vi "Phaeron App Template.vi"() -> ()   [LabVIEW 2013]
uses:
  <vilib>/Utility/miscctls.llb/LVPointTypeDef.ctl
  <vilib>/NI/AMC/Read Next Message.vi
  <vilib>/NI/AMC/Create Single Message.vi
  <vilib>/NI/AMC/Update Message Routing Info.vi
  <vilib>/NI/AMC/Read Termination Message.vi
  <vilib>/NI/AMC/Send Message.vi
  <vilib>/NI/AMC/Globals.vi
  <vilib>/NI/AMC/AMC.lvlib
  <vilib>/Phaeron, Inc/JSON/LV JSON.lvlib
panel:
  in  "Stop Loops":bool
  in  "Exit":bool
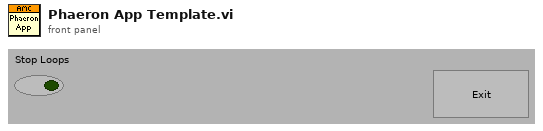
[diagram p1: front panel]
types:
  T1 = typedef "AMC.lvlib/Message Queue.ctl" = refnum<queue>
  T2 = typedef "LVPointTypeDef.ctl" = cluster{"Horizontal":i16, "Vertical":i16}
  T3 = typedef "LVRectTypeDef.ctl" = cluster{"Left":i16, "Top":i16, "Right":i16, "Bottom":i16}
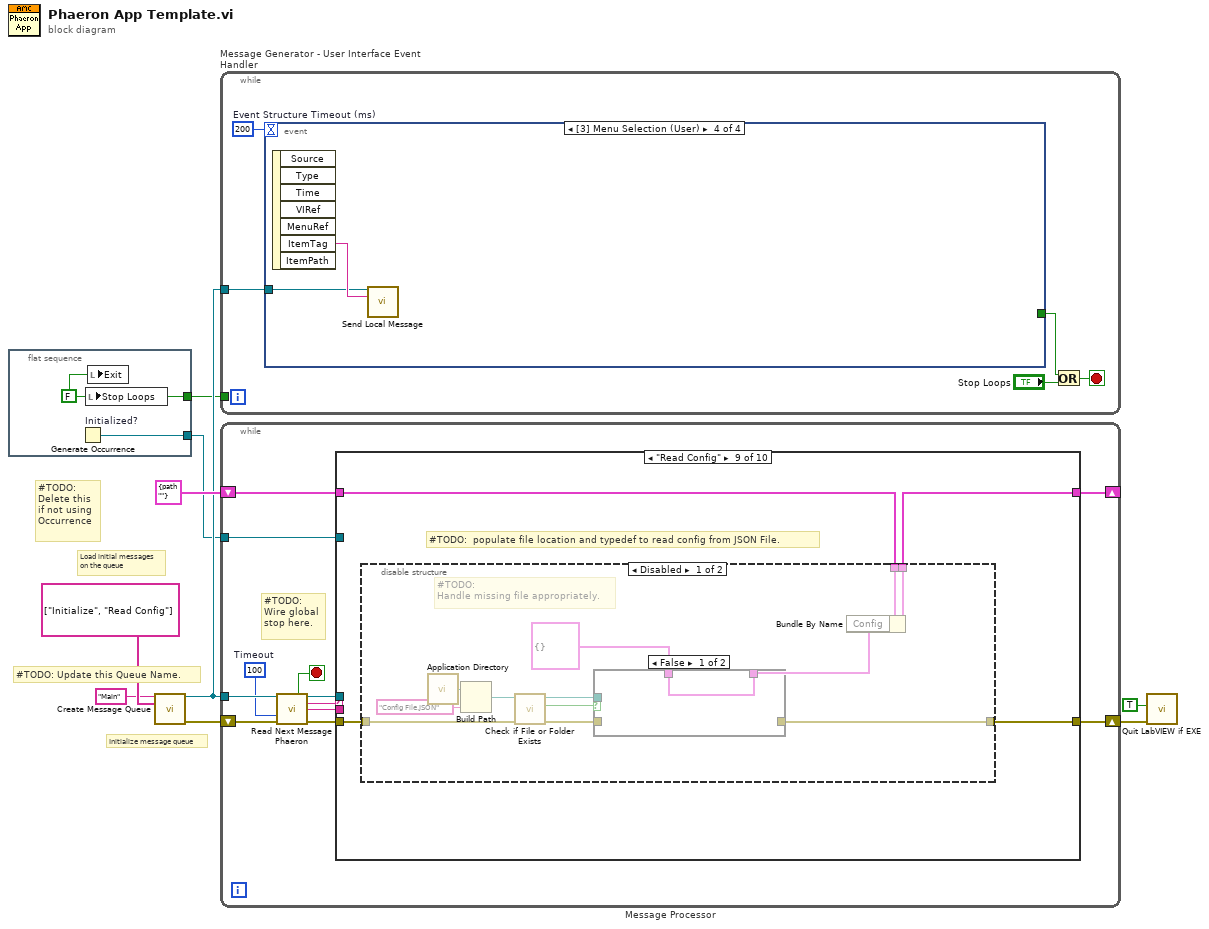
[diagram p0: block diagram]
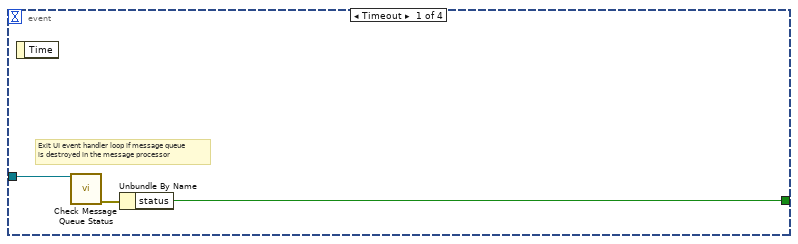
[diagram p2: hidden frame]
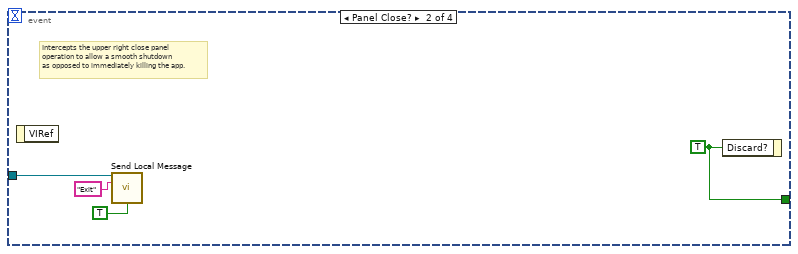
[diagram p3: hidden frame]
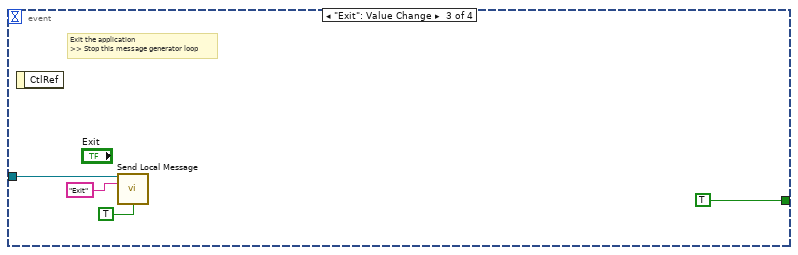
[diagram p4: hidden frame]
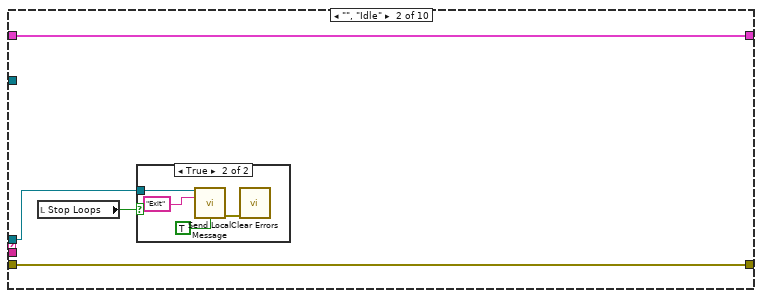
[diagram p6: hidden frame]
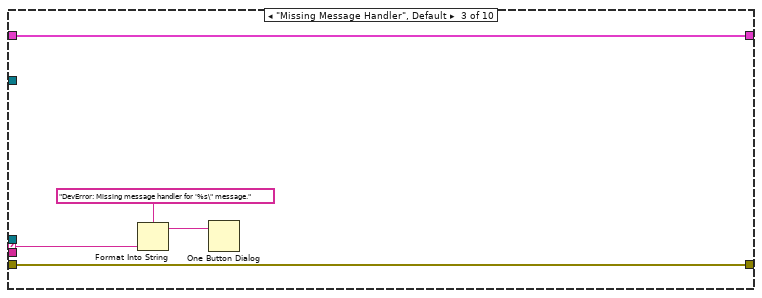
[diagram p8: hidden frame]
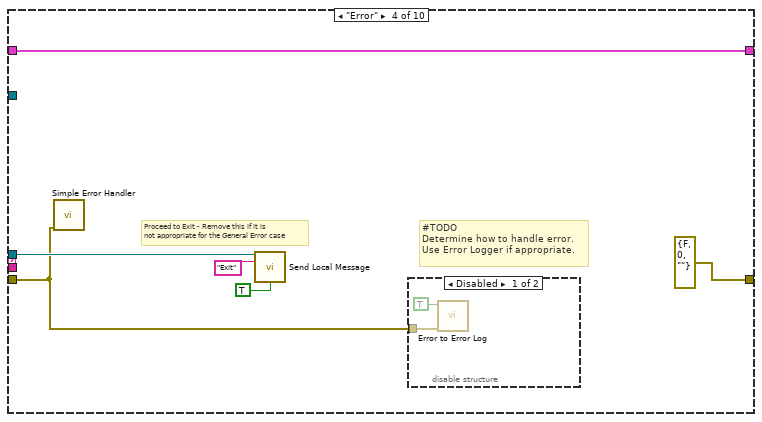
[diagram p9: hidden frame]
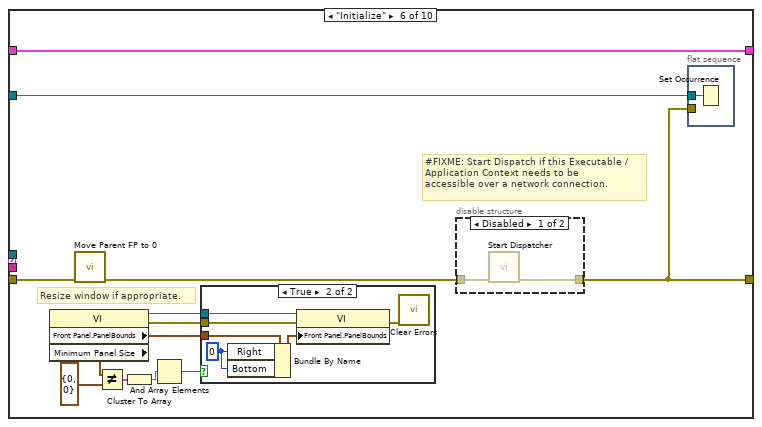
[diagram p12: hidden frame]
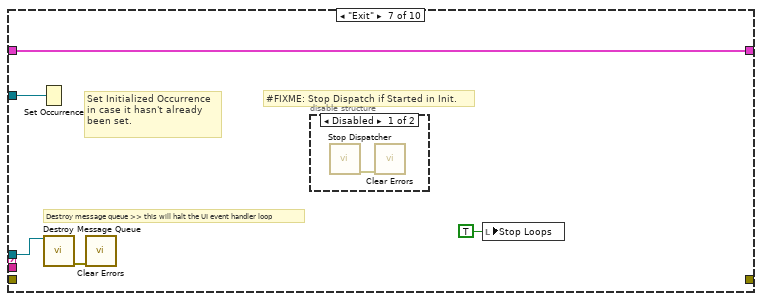
[diagram p15: hidden frame]
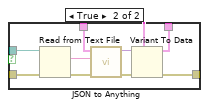
[diagram p18: hidden frame]
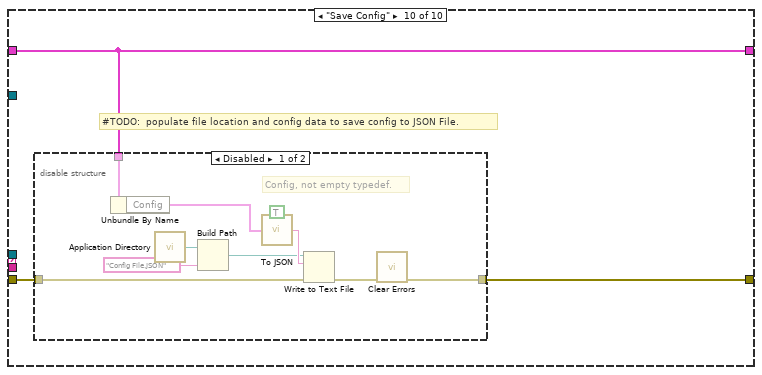
[diagram p20: hidden frame]
diagram:
  # "#TODO:\nDelete this\nif not using\nOccurrence"
  # "#TODO: Update this Queue Name."
  # "Initialize message queue"
  # "Load initial messages\non the queue"
  n1 = flat-sequence {
    tunnel: [w10] -> w4
    tunnel: [w11] -> w1
    frame #0 {
      w10 = FALSE ("Stop Loops")
      n2 = Generate Occurrence "Initialized?"() -> (w11:refnum<k4>)
      n3 = local write "Stop Loops"(w10) -> ()
      n4 = local write "Exit"(w10) -> ()
    }
  }
  n5 = call <vilib>:"Create Message Queue.vi"("message queue name"="Main", "initial message names"=string[] ["Initialize", "Read Config"]) -> ("message queue out"=w7:T1, "error out"=w8:errorcluster)  [unwired: 12 in]
  n6 = while "Message Generator - User Interface Event Handler" {
    tunnel: w7 -> [w14]
    tunnel: w4 -> [_]
    stop <- w13 stop-if-true
    w16 = 200  # Event Structure Timeout (ms)
    n7 = event shown="[3] Menu Selection (User)" {
      selector: _ -> [_ _ _ _]
      dyn-events: _ -> [_ _ _ _]
      timeout: w16 -> [_ _ _ _]
      tunnel: [w17 w20 TRUE ("Discard?") _] -> w15
      tunnel: w14 -> [w18 w22 w25 w28]
      event Timeout {
        # "Exit UI event handler loop if message queue\nis destroyed in the message processor"
        n8 = event-data() -> ()  [unwired: 2 out]
        n9 = call <vilib>:"Check Message Queue Status.vi"("message queue in"=w18) -> ("error out"=w19:errorcluster)  [unwired: 10 in, 4 out]
        n10 = Unbundle By Name(w19) -> ("status"=w17:bool)
      }
      event Panel Close? {
        w20 = TRUE ("Discard?")
        # "Intercepts the upper right close panel\noperation to allow a smooth shutdown\nas opposed to immediately killing the app."
        n11 = event-data() -> ()  [unwired: 2 out]
        n12 = call <vilib>:"Send Local Message.vi"("message queue in"=w22, "message name"="Exit", "priority message (F)"=TRUE) -> ()  [unwired: 10 in, 3 out]
        n13 = event-data("Discard?"=w20) -> ()  [unwired: 1 in, 1 out]
      }
      event "Exit": Value Change {
        # "Exit the application\n>> Stop this message generator loop"
        n14 = event-data() -> ()  [unwired: 2 out]
        n15 = call <vilib>:"Send Local Message.vi"("message queue in"=w25, "message name"="Exit", "priority message (F)"=TRUE) -> ()  [unwired: 10 in, 3 out]
      }
      event Menu Selection (User) {
        n16 = event-data() -> ("ItemTag"=w29:string)  [unwired: 7 out]
        n17 = call <vilib>:"Send Local Message.vi"("message queue in"=w28, "message name"=w29) -> ()  [unwired: 11 in, 3 out]
      }
    }
    n18 = Or(x=w15, y="Stop Loops") -> (x .or. y?=w13:bool)
  }
  n19 = while "Message Processor" {
    shift-left: w8 -> [w35]
    shift-right: [w39] -> w3
    tunnel: w7 -> [w36]
    shift-left: cluster{"CurrentFile":path} {"CurrentFile"=path ""} ("State Variables") -> [w41]
    shift-right: [w40] -> _
    tunnel: w1 -> [w30]
    stop <- w38 stop-if-true
    w31 = 100  # Timeout
    # "#TODO:\nWire global\nstop here."
    n20 = call "Read Next Message Phaeron.vi"("message queue in"=w36, "timeout (1 ms)"=w31, "error in"=w35) -> ("exit process?"=w38:bool, "message queue out"=w37:T1, "message name"=w33:string, "message value"=w32:string, "error out"=w34:errorcluster)  [unwired: 5 in, 3 out]
    n21 = case shown="\"Read Config\"" w33 {
      selector: w33 -> [_ _ w54 _ _ _ _ _ _ _]
      tunnel: [w43 w47 w56 w62 w66 w79 w94 w97 w98 w126] -> w40
      tunnel: w41 -> [w43 w47 w56 w62 w66 w79 w94 w97 w99 w126]
      tunnel: w37 -> [_ w45 _ w60 _ _ w93 _ _ _]
      tunnel: w34 -> [w42 w46 w55 w57 w65 w78 _ w96 w101 w128]
      tunnel: [w42 w46 w55 errorcluster {"status"=FALSE, "code"=0, "source"=""} ("error out") w65 w75 _ w96 w100 w127] -> w39
      tunnel: w32 -> [_ _ _ _ _ _ _ _ _ _]
      tunnel: w30 -> [_ _ _ _ _ w76 w90 _ _ _]
      frame "---------- Framework Operations ----------" {
      }
      frame "", "Idle" {
        n22 = local read "Stop Loops"() -> (w44:bool)
        n23 = case shown="True" w44 {
          tunnel: w45 -> [_ w48]
          frame False {
          }
          frame True {
            n24 = call <vilib>:"Send Local Message.vi"("message queue in"=w48, "message name"="Exit", "priority message (F)"=TRUE) -> ("error out"=w49:errorcluster)  [unwired: 10 in, 2 out]
            n25 = call <vilib>:"Clear Errors.vi"("error in (no error)"=w49) -> ()  [unwired: 6 in, 1 out]
          }
        }
      }
      frame "Missing Message Handler", Default {
        n26 = Format Into String(format string="DevError: Missing message handler for '%s\" message." ("message"), w54) -> (resulting string=w52:string)  [unwired: 2 in, 1 out]
        n27 = One Button Dialog(message=w52) -> ()  [unwired: 2 out]
      }
      frame "Error" {
        # "#TODO\nDetermine how to handle error.\nUse Error Logger if appropriate."
        # "Proceed to Exit - Remove this if it is\nnot appropriate for the General Error case"
        n28 = call <vilib>:"Simple Error Handler.vi"("error in (no error)"=w57) -> ()  [unwired: 1 in, 8 out]
        n29 = call <vilib>:"Send Local Message.vi"("message queue in"=w60, "message name"="Exit", "priority message (F)"=TRUE) -> ()  [unwired: 10 in, 3 out]
        n30 = disable-structure shown="Disabled" {
          disable-tunnel: w57 -> [w64 _]
          frame Disabled {
            n31 = call "Error to Error Log.vi"("error in (no error)"=w64, "Clear?"=TRUE) -> ()  [unwired: 8 in, 2 out]
          }
          frame Enabled {
          }
        }
      }
      frame "---------- Generic Operations ----------" {
      }
      frame "Initialize" {
        # "Resize window if appropriate."
        # "#FIXME: Start Dispatch if this Executable /\nApplication Context needs to be\naccessible over a network connection."
        n32 = property class="VI"() -> (reference out=w72:refnum<vi>, error out=w73:errorcluster, "Front Panel.PanelBounds"=w74:T3, "Minimum Panel Size"=w70:T2)  [unwired: 2 in]
        n33 = call "Move Parent FP to 0.vi"("error in"=w78) -> ("error out"=w77:errorcluster)  [unwired: 10 in]
        n34 = Not Equal?(x=w70, y=T2 {"Horizontal"=0, "Vertical"=0} ("Front Panel Window:Minimum Size")) -> (x != y?=w69:cluster{"Horizontal":bool, "Vertical":bool})
        n35 = Cluster To Array(cluster=w69) -> (array=w68:bool[])
        n36 = And Array Elements(Boolean array=w68) -> (logical AND=w67:bool)
        n37 = case shown="True" w67 {
          tunnel: w74 -> [_ w83]
          tunnel: w73 -> [_ w82]
          tunnel: w72 -> [_ w81]
          frame False {
          }
          frame True {
            w85 = i16 0 ("Right")
            n38 = Bundle By Name(cluster=w83, "Right"=w85, "Bottom"=w85) -> (w84:T3)
            n39 = property class="VI"(reference=w81, error in=w82, "Front Panel.PanelBounds"=w84) -> (error out=w80:errorcluster)  [unwired: 1 out]
            n40 = call <vilib>:"Clear Errors.vi"("error in (no error)"=w80) -> ()  [unwired: 6 in, 1 out]
          }
        }
        n41 = disable-structure shown="Disabled" {
          disable-tunnel: w77 -> [w88 w89]
          disable-tunnel: [w87 w89] -> w75
          frame Disabled {
            n42 = call <vilib>:"Start Dispatcher.vi"("error in"=w88) -> ("error out"=w87:errorcluster)  [unwired: 12 in, 2 out]
          }
          frame Enabled {
          }
        }
        n43 = flat-sequence {
          tunnel: w76 -> [w86]
          tunnel: w75 -> [_]
          frame #0 {
            n44 = Set Occurrence(w86) -> ()
          }
        }
      }
      frame "Exit" {
        # "Set Initialized Occurrence\nin case it hasn't already\nbeen set."
        # "#FIXME: Stop Dispatch if Started in Init."
        # "Destroy message queue >> this will halt the UI event handler loop"
        n45 = Set Occurrence(w90) -> ()
        n46 = call <vilib>:"Destroy Message Queue.vi"("message queue in"=w93) -> ("error out"=w92:errorcluster)  [unwired: 12 in, 2 out]
        n47 = call <vilib>:"Clear Errors.vi"("error in (no error)"=w92) -> ()  [unwired: 6 in, 1 out]
        n48 = disable-structure shown="Disabled" {
          frame Disabled {
            n49 = call <vilib>:"Stop Dispatcher.vi"() -> ("error out"=w95:errorcluster)  [unwired: 15 in]
            n50 = call <vilib>:"Clear Errors.vi"("error in (no error)"=w95) -> ()  [unwired: 6 in, 1 out]
          }
          frame Enabled {
          }
        }
        n51 = local write "Stop Loops"(TRUE ("Stop Loops")) -> ()
      }
      frame "---------- Application Operations ----------" {
      }
      frame "Read Config" {
        # "#TODO:  populate file location and typedef to read config from JSON File."
        n52 = disable-structure shown="Disabled" {
          disable-tunnel: w101 -> [w107 w125]
          disable-tunnel: [w103 w125] -> w100
          disable-tunnel: w99 -> [w110 w124]
          disable-tunnel: [w109 w124] -> w98
          frame Disabled {
            # "#TODO:\nHandle missing file appropriately."
            n53 = call <vilib>:"Application Directory.vi"() -> ("Application Directory"=w112:path)
            n54 = Build Path(base path=w112, name or relative path="Config File.JSON") -> (appended path=w106:path)
            n55 = call <vilib>:"Check if File or Folder Exists.vi"("error in (no error)"=w107, "path"=w106) -> ("error out"=w104:errorcluster, "file or folder exists?"=w102:bool, "dup path"=w105:path)  [unwired: 7 in]
            n56 = case shown="False" w102 {
              tunnel: cluster{} {} -> [w114 w119]
              tunnel: [w114 w118] -> w108
              tunnel: w105 -> [_ w117]
              tunnel: w104 -> [_ w116]
              tunnel: [_ w115] -> w103
              frame False {
              }
              frame True {
                n57 = Read from Text File(file (use dialog)=w117, error in=w116) -> (text=w121:string, error out=w120:errorcluster)  [unwired: 2 in, 2 out]
                n58 = call <vilib>:"JSON to Anything.vi"("error in (no error)"=w120, "JSON Object"=w121, "Type"=w119) -> ("error out"=w123:errorcluster, "Variant"=w122:variant)  [unwired: 5 in, 2 out]
                n59 = Variant To Data(error in=w123, type=w119, Variant=w122) -> (data=w118:cluster{}, error out=w115:errorcluster)
              }
            }
            n60 = Bundle By Name(cluster=w110, "Config"=w108) -> (w109:cluster{"CurrentFile":path})
          }
          frame Enabled {
          }
        }
      }
      frame "Save Config" {
        # "#TODO:  populate file location and config data to save config to JSON File."
        n61 = disable-structure shown="Disabled" {
          disable-tunnel: w128 -> [w133 w139]
          disable-tunnel: [w138 w139] -> w127
          disable-tunnel: w126 -> [w130 _]
          frame Disabled {
            # "Config, not empty typedef."
            n62 = Unbundle By Name(w130) -> ("Config"=w129:cluster{})
            n63 = call <vilib>:"Application Directory.vi"() -> ("Application Directory"=w137:path)
            n64 = Build Path(base path=w137, name or relative path="Config File.JSON") -> (appended path=w131:path)
            n65 = call <vilib>:"To JSON.vi"("Anything"=w129, "Pretty Print (F)"=TRUE) -> ("JSON"=w135:string)
            n66 = Write to Text File(file (use dialog)=w131, text=w135, error in=w133) -> (error out=w132:errorcluster)  [unwired: 1 in, 2 out]
            n67 = call <vilib>:"Clear Errors.vi"("error in (no error)"=w132) -> ("error out"=w138:errorcluster)  [unwired: 6 in]
          }
          frame Enabled {
          }
        }
      }
    }
  }
  n68 = call "Quit LabVIEW if EXE.vi"("error in (no error)"=w3, "Quit LabVIEW?"=TRUE) -> ()  [unwired: 9 in, 1 out]
